vi "send data to imaging mode.vi"(8 "error in (no error)":errorcluster, 9 "Amplitude2":dbl, 10 "Amplitude1":dbl, 11 "Tomo in":refnum<class "Tomo.lvclass">) -> (0 "error out":errorcluster, 3 "Tomo out":refnum<class "Tomo.lvclass">)   [LabVIEW 2012, in "Tomo.lvclass"]
uses:
  Tomo.lvclass
  <vilib>/Distrio/Murmex/Murmex/update_cluster.ctl
  <vilib>/Distrio/Murmex/StartMessage/StartMessage.lvclass
  <vilib>/Distrio/Murmex/StartMessage/run mode enum.ctl
  Tomo.lvclass/Tomo.ctl
  <vilib>/Distrio/Murmex/Murmex/Murmex.lvclass
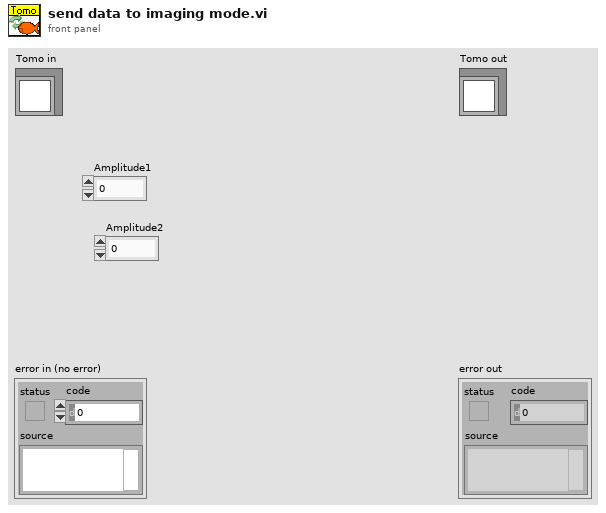
[diagram p1: front panel]
types:
  T1 = typedef "Murmex.lvlib/StartMessage.lvclass/run mode enum.ctl" = enum16{"infinite", "finite"}
  T2 = typedef "Murmex.lvlib/Murmex.lvclass/update_cluster.ctl" = cluster{"target ID":string, "key chains":string[], "values":variant[]}
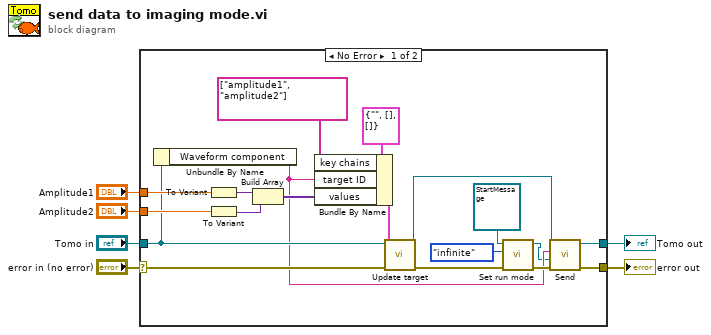
[diagram p0: block diagram]
diagram:
  n1 = case shown="No Error" "error in (no error)" {
    selector: "error in (no error)" -> [w17 w27]
    tunnel: [w11 w27] -> w5
    tunnel: [w7 w26] -> w3
    tunnel: "Tomo in" -> [w16 w26]
    tunnel: "Amplitude1" -> [w19 _]
    tunnel: "Amplitude2" -> [w18 _]
    frame No Error {
      n2 = Unbundle By Name(w16) -> ("Waveform component"=w10:string)
      n3 = To Variant(anything=w19) -> (Variant=w21:variant)
      n4 = To Variant(anything=w18) -> (Variant=w25:variant)
      n5 = Build Array(w21, w25) -> (w22:variant[])
      n6 = Bundle By Name(cluster=T2 {"target ID"="", "key chains"=[], "values"=[]} ("update cluster"), "key chains"=string[] ["amplitude1", "amplitude2"], "target ID"=w10, "values"=w22) -> (w23:T2)
      n7 = call <vilib>:"Update target.vi"("error in (no error)"=w17, "update cluster"=w23, "MurmexBase in"=w16) -> ("error out"=w13:errorcluster, "MurmexBase out"=w8:refnum<class "Tomo.lvclass">)  [unwired: 7 in]
      n8 = call <vilib>:"Set run mode.vi"("error in (no error)"=w13, "run mode"=run_mode_enum."infinite", "StartMessage in"=refnum<class "StartMessage.lvclass"> refnum ("Message in")) -> ("error out"=w12:errorcluster, "StartMessage out"=w9:refnum<class "StartMessage.lvclass">)  [unwired: 7 in]
      n9 = call <vilib>:"Send.vi"("error in (no error)"=w12, "Message"=w9, "recipient"=w10, "Murmex in"=w8) -> ("error out"=w11:errorcluster, "Murmex out"=w7:refnum<class "Tomo.lvclass">)  [unwired: 6 in]
    }
    frame Error {
    }
  }
  "error out" <- w5
  "Tomo out" <- w3
